vi "generatore_rettangolare_0_1.vi"(0 "f0 (frequenza base) [Hz]":dbl min=0.0, 1 "Ap (ampiezza di picco)":dbl min=0.0, 2 "Tc (periodo di campionamento) [s]":dbl min=0.0, 3 "Ta (tempo di analisi) [s]":dbl min=0.0, 4 "Duty Cycle (onda rettangolare)":dbl min=0.0 max=1.0, 5 "Phi (fase iniziale) [rad]":dbl, 8 "DC Offset":dbl) -> (7 "Waveform Graph":waveform(dbl)(graph))   [LabVIEW 2009]
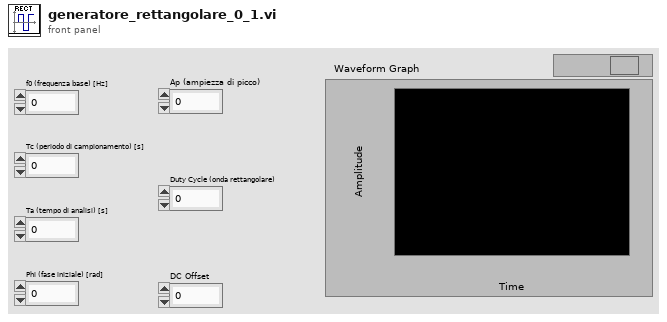
[diagram p1: front panel]
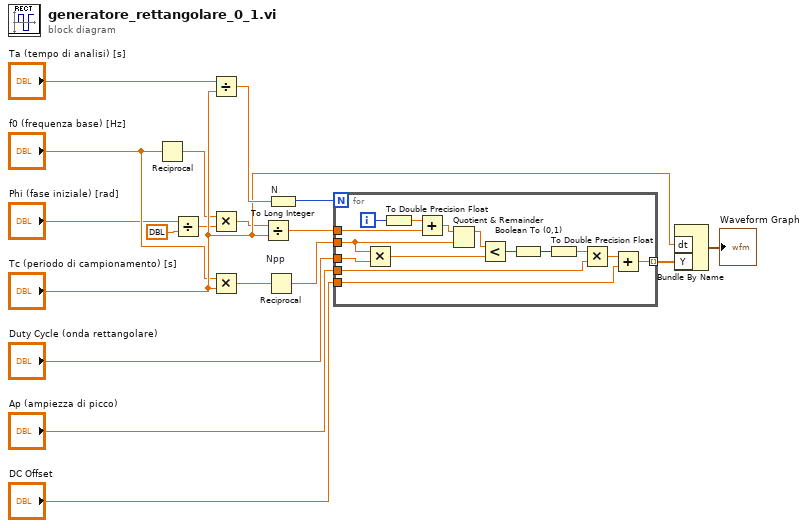
[diagram p0: block diagram]
diagram:
  n1 = Reciprocal(x="f0 (frequenza base) [Hz]") -> (1/x=w3:dbl)
  n2 = Divide(x="Phi (fase iniziale) [rad]", y=dbl ?) -> (x/y=w4:dbl)
  n3 = Divide(x="Ta (tempo di analisi) [s]", y="Tc (periodo di campionamento) [s]") -> (x/y=w12:dbl)
  n4 = Multiply(x=w3, y=w4) -> (x*y=w2:dbl)
  n5 = Multiply(x="f0 (frequenza base) [Hz]", y="Tc (periodo di campionamento) [s]") -> (x*y=w17:dbl)
  n6 = Divide(x=w2, y="Tc (periodo di campionamento) [s]") -> (x/y=w1:dbl)
  n7 = Reciprocal "Npp"(x=w17) -> (1/x=w18:dbl)
  n8 = To Long Integer "N"(number=w12) -> (32bit integer=w13:i32)
  n9 = for {
    N: w13 -> [_]
    tunnel: "DC Offset" -> [w33]
    tunnel: "Ap (ampiezza di picco)" -> [w21]
    tunnel: "Duty Cycle (onda rettangolare)" -> [w31]
    tunnel: [w32] -> w10 mode=indexing
    tunnel: w18 -> [w30]
    tunnel: w1 -> [w19]
    i -> [w29]
    n10 = Multiply(x=w30, y=w31) -> (x*y=w25:dbl)
    n11 = To Double Precision Float(number=w29) -> (double precision float=w28:dbl)
    n12 = Add(x=w28, y=w19) -> (x+y=w27:dbl)
    n13 = Quotient & Remainder(x=w27, y=w30) -> (x-y*floor(x/y)=w26:dbl)  [unwired: 1 out]
    n14 = Less?(x=w26, y=w25) -> (x < y?=w24:bool)
    n15 = Boolean To (0,1)(Boolean=w24) -> (0, 1=w23:i16)
    n16 = To Double Precision Float(number=w23) -> (double precision float=w22:dbl)
    n17 = Multiply(x=w22, y=w21) -> (x*y=w20:dbl)
    n18 = Add(x=w20, y=w33) -> (x+y=w32:dbl)
  }
  n19 = Bundle By Name("dt"="Tc (periodo di campionamento) [s]", "Y"=w10) -> (→"Waveform Graph":waveform(dbl))  [unwired: 1 in]
